vi "Add Context.vi"(4 "MultiErrors in":refnum<class "MultiErrors.lvclass">, 5 "Context":string) -> (6 "Added Context":refnum<class "MultiErrors.lvclass">, 7 "Original Context":refnum<class "MultiErrors.lvclass">)   [LabVIEW 2020, in "Volatus.lvlib" / "MultiErrors.lvclass"]
uses:
  MultiErrors.lvclass
  MultiErrors.lvclass/MultiErrors.ctl
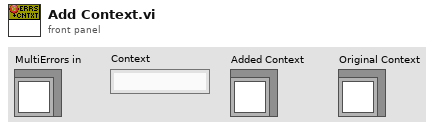
[diagram p1: front panel]
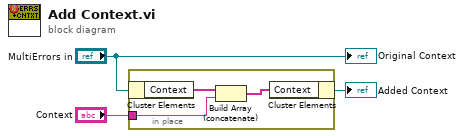
[diagram p0: block diagram]
diagram:
  n1 = in-place {
    in-place-border: "Context" -> [w5]
    n2 = in-place-cluster #1("MultiErrors in") -> ("Context"=w6:string[])
    n3 = Build Array (concatenate)(w6, w5) -> (w4:string[])
    n4 = in-place-cluster #1("Context"=w4) -> (→"Added Context":refnum<class "MultiErrors.lvclass">)
  }
  "Original Context" <- "MultiErrors in"
